vi "Measurement Root Path.vi"(8 "error in (no error)":errorcluster, 10 "Operation (Get)":enum16{"Get", "Set"}(ring), 11 "Measurement Library Path":path) -> (0 "error out":errorcluster, 3 "Measurement Library Path out":path)   [LabVIEW 2020, in "MeasurementLink Measurement Server.lvlib"]
uses:
  MeasurementLink Measurement Server.lvlib
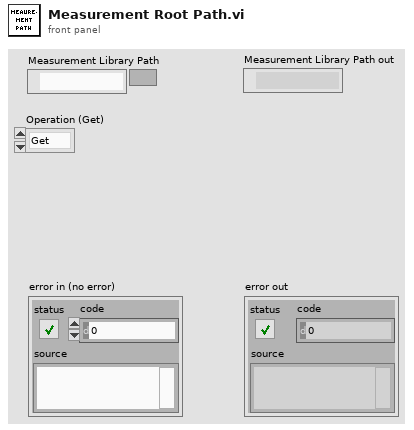
[diagram p1: front panel]
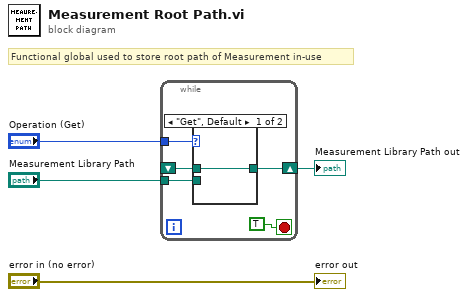
[diagram p0: block diagram]
diagram:
  # "Functional global used to store root path of Measurement in-use"
  n1 = while {
    tunnel: "Operation (Get)" -> [w8]
    tunnel: "Measurement Library Path" -> [w6]
    shift-right: [w7] -> w2
    shift-left: _ -> [w5]
    stop <- TRUE stop-if-true
    n2 = case shown="\"Get\", Default" w8 {
      tunnel: [w10 w11] -> w7
      tunnel: w6 -> [_ w11]
      tunnel: w5 -> [w10 _]
      frame "Get", Default {
      }
      frame "Set" {
      }
    }
  }
  "Measurement Library Path out" <- w2
  "error out" <- "error in (no error)"
